vi "NewDax_ReadGains.vi"(10 "Ch Option":enum16{"Gains", "Delays", "Slope", "Enable"}(ring), 11 "Daxsonics VISA":refnum<visa-resource-name>="COM8") -> (0 "Array":i32[][](array[numeric]), 2 "Values Out":i32[](array[numeric]))   [LabVIEW 2022 SP3]
uses:
  Daxsonics_Pulsers.ctl
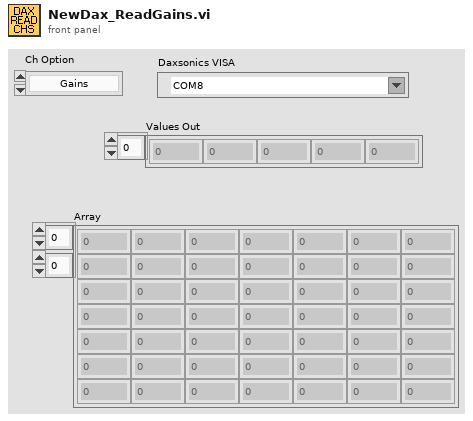
[diagram p1: front panel]
types:
  T1 = typedef "Daxsonics_Pulsers.ctl" = enum16{"BP1", "BP2_A", "BP2_B", "10ERS8", "New2021"}
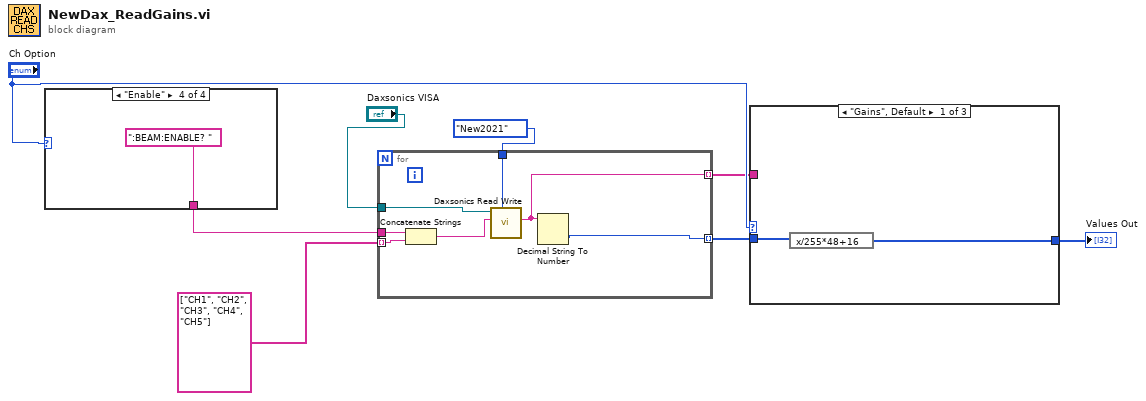
[diagram p0: block diagram]
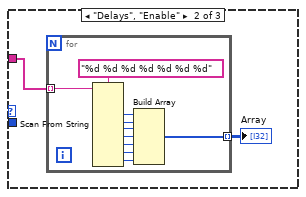
[diagram p2: hidden frame]
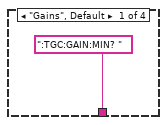
[diagram p4: hidden frame]
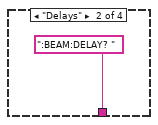
[diagram p5: hidden frame]
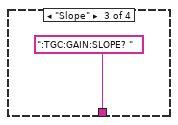
[diagram p6: hidden frame]
diagram:
  n1 = case shown="\"Enable\"" "Ch Option" {
    tunnel: [":TGC:GAIN:MIN? " ":BEAM:DELAY? " ":TGC:GAIN:SLOPE? " ":BEAM:ENABLE? "] -> w8
    frame "Gains", Default {
    }
    frame "Delays" {
    }
    frame "Slope" {
    }
    frame "Enable" {
    }
  }
  n2 = for {
    tunnel: "Daxsonics VISA" -> [w19]
    tunnel: [w14] -> w4 mode=indexing
    tunnel: w8 -> [w18]
    tunnel: string[] ["CH1", "CH2", "CH3", "CH4", "CH5"] -> [w17] mode=indexing
    tunnel: [w15] -> w2 mode=indexing
    tunnel: Daxsonics_Pulsers."New2021" ("Daxsonics Name") -> [w13]
    n3 = Concatenate Strings(w18, w17) -> (w16:string)
    n4 = call "Daxsonics Read Write.vi"("Daxsonics Name"=w13, "write buffer"=w16, "VISA resource name"=w19) -> ("read buffer"=w15:string)  [unwired: 6 in, 2 out]
    n5 = Decimal String To Number(string=w15) -> (number=w14:i32)  [unwired: 2 in, 1 out]
  }
  n6 = case shown="\"Gains\", Default" "Ch Option" {
    tunnel: w4 -> [w21 _ w34]
    tunnel: [w20 _ w34] -> w3
    tunnel: w2 -> [_ w23 _]
    frame "Gains", Default {
      n7 = expression code="x/255*48+16"(w21) -> (w20:i32[])
    }
    frame "Delays", "Enable" {
      n8 = for {
        tunnel: w23 -> [w26] mode=indexing
        tunnel: [w24] -> w22 mode=indexing
        n9 = Scan From String(format string="%d %d %d %d %d %d %d", input string=w26) -> (output 1=w27:i32, output 2=w28:i32, output 3=w29:i32, output 4=w30:i32, output 5=w31:i32, output 6=w32:i32, output 7=w33:i32)  [unwired: 9 in, 3 out]
        n10 = Build Array(w27, w28, w29, w30, w31, w32, w33) -> (w24:i32[])
      }
      "Array" <- w22
    }
    frame "Slope" {
    }
  }
  "Values Out" <- w3
